vi "FABR-Append Stimulus Queue.vi"(0 "Runtime in":T2, 7 "SCL in":cluster{T1[]}[](array[cluster]), 11 "error in (no error)":errorcluster) -> (4 "Runtime out":T2, 8 "SCL out":cluster{T1[]}[](array[cluster]), 15 "error out":errorcluster)   [LabVIEW 2020]
uses:
  Typedefs/FABR-Runtime Data.ctl
  Typedefs/FABR-Stimulus Ticket.ctl
  Typedefs/FABR-Order.ctl
  Typedefs/FABR-Stimulus Condition.ctl
  debe6c45-fa08-4a77-9124-1a41b649b6a5.vi
  epl-vi-lib/Utility VIs/Math VIs/Math-Uniform Random Number (I32, 1D).vi
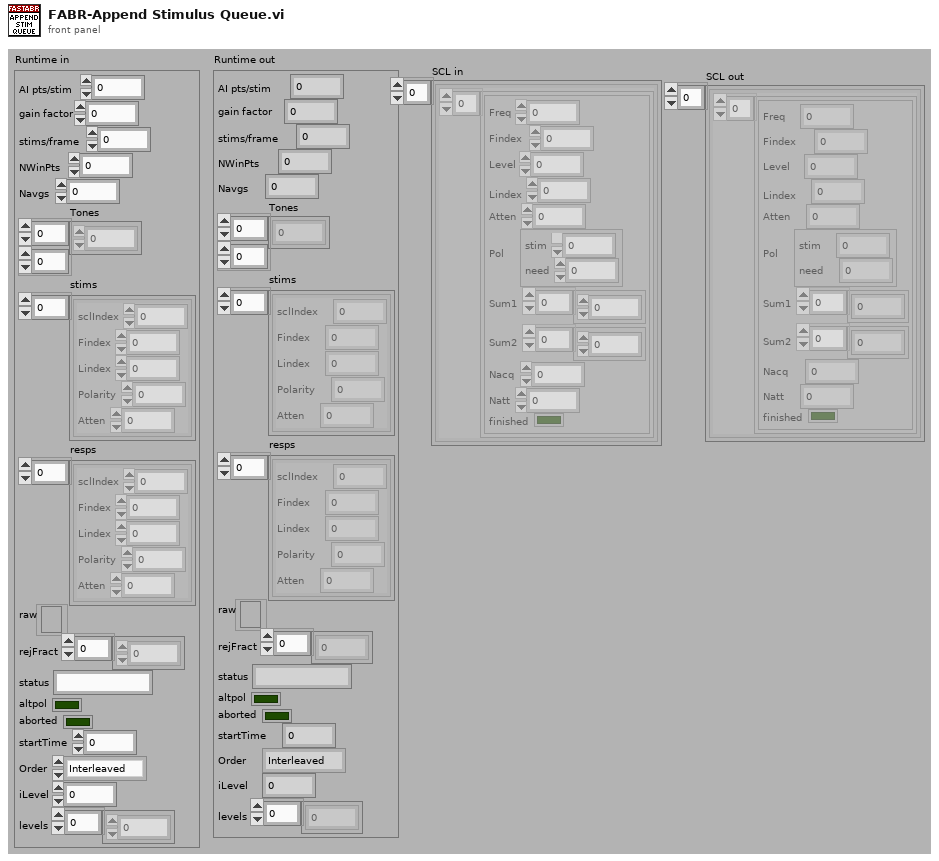
[diagram p1: front panel]
types:
  T1 = typedef "FABR-Stimulus Condition.ctl" = cluster{"Freq":dbl, "Findex":i32, "Level":dbl, "Lindex":i32, "Atten":dbl, "Pol":cluster{"stim":i32, "need":i32}, "Sum1":dbl[], "Sum2":dbl[], "Nacq":i32, "Natt":i32, "finished":bool}
  T2 = typedef "FABR-Runtime Data.ctl" = cluster{"AI pts/stim":i32, "gain factor":dbl, "stims/frame":i32, "NWinPts":i32, "Navgs":i32, "Tones":dbl[][], "stims":T3[], "resps":T3[], "raw":refnum<file>, "rejFract":dbl[], "status":string, "altpol":bool, "aborted":bool, "startTime":dbl, "Order":T4, "iLevel":i32, "levels":dbl[]}
  T3 = typedef "FABR-Stimulus Ticket.ctl" = cluster{"sclIndex":i32, "Findex":i32, "Lindex":i32, "Polarity":i32, "Atten":dbl}
  T4 = typedef "FABR-Order.ctl" = enum16{"Interleaved", "Stepped level"}
  T5 = cluster{i32, "Findex":i32, "Lindex":i32, "stim":i32, "Atten":dbl}
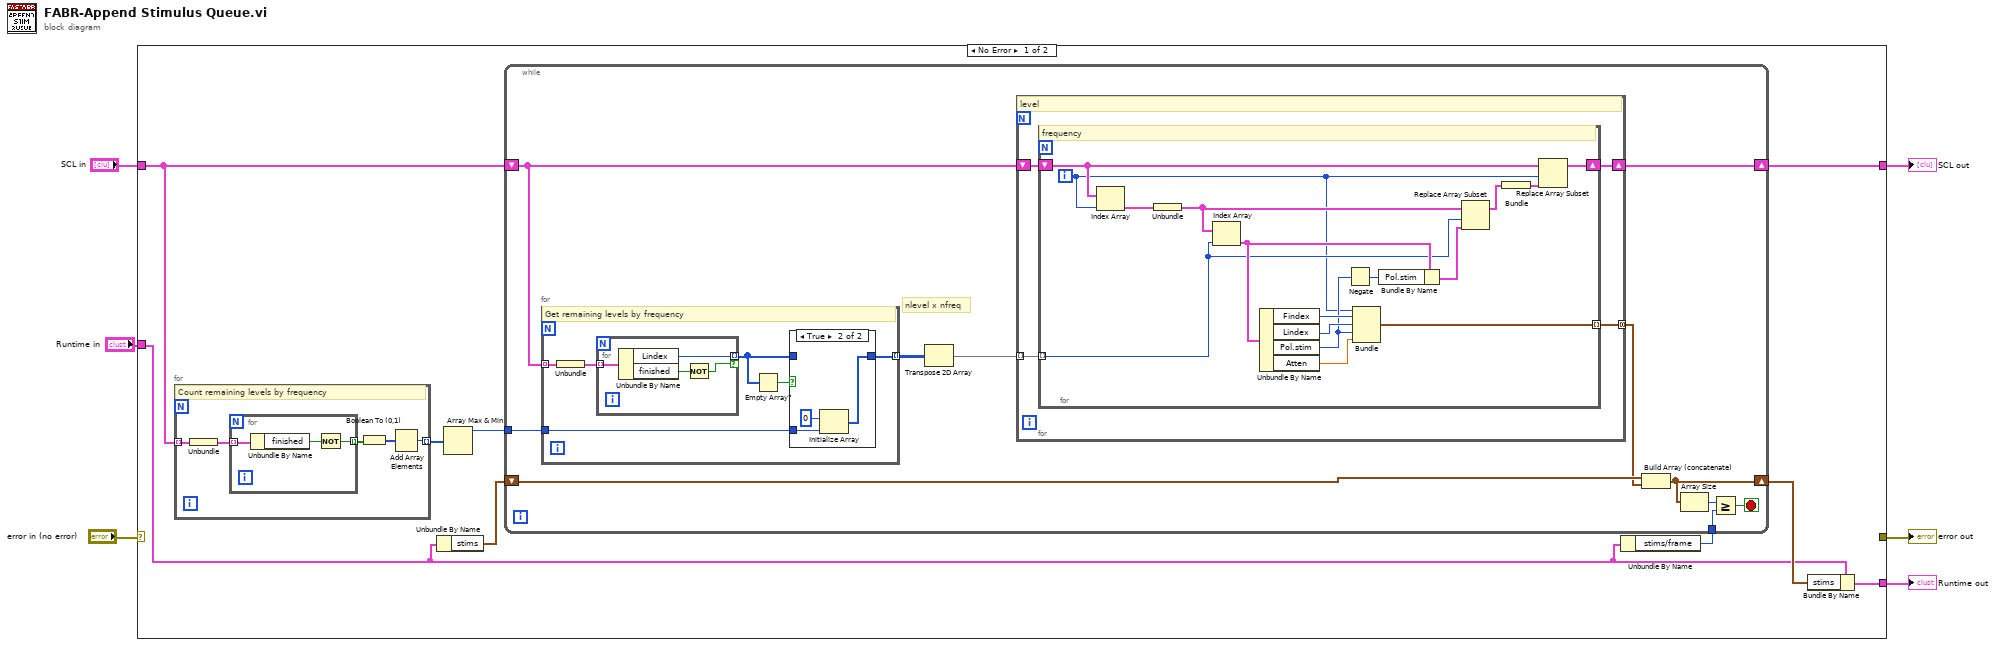
[diagram p0: block diagram]
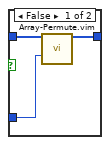
[diagram p2: hidden frame]
diagram:
  n1 = case shown="No Error" "error in (no error)" {
    selector: "error in (no error)" -> [_ w73]
    tunnel: [_ w73] -> w6
    tunnel: "Runtime in" -> [w8 w72]
    tunnel: [w13 w72] -> w4
    tunnel: "SCL in" -> [w14 w71]
    tunnel: [w12 w71] -> w1
    frame No Error {
      n2 = for {
        tunnel: w14 -> [w67] mode=indexing
        tunnel: [w63] -> w15 mode=indexing
        # "Count remaining levels by frequency"
        n3 = Unbundle(w67) -> (w66:T1[])
        n4 = for {
          tunnel: w66 -> [w70] mode=indexing
          tunnel: [w68] -> w64 mode=indexing
          n5 = Unbundle By Name(w70) -> ("finished"=w69:bool)
          n6 = Not(x=w69) -> (.not. x?=w68:bool)
        }
        n7 = Boolean To (0,1)(Boolean=w64) -> (0, 1=w65:i16[])
        n8 = Add Array Elements(numeric array=w65) -> (sum=w63:i16)
      }
      n9 = Unbundle By Name(w8) -> ("stims"=w10:T3[])
      n10 = Array Max & Min(array=w15) -> (max value=w11:i16)  [unwired: 3 out]
      n11 = Unbundle By Name(w8) -> ("stims/frame"=w7:i32)
      n12 = while {
        tunnel: w7 -> [w22]
        tunnel: w11 -> [w21]
        shift-right: [w23] -> w12
        shift-left: w14 -> [w25]
        shift-right: [w19] -> w9
        shift-left: w10 -> [w20]
        stop <- w16 stop-if-true
        # "nlevel x nfreq"
        n13 = for {
          tunnel: w25 -> [w52] mode=indexing
          tunnel: w21 -> [w50]
          tunnel: [w49] -> w26 mode=indexing
          # "Get remaining levels by frequency"
          n14 = Unbundle(w52) -> (w51:T1[])
          n15 = for {
            tunnel: w51 -> [w62] mode=indexing
            tunnel: [w60] -> w48 mode=indexing if=w59
            n16 = Unbundle By Name(w62) -> ("Lindex"=w60:i32, "finished"=w61:bool)
            n17 = Not(x=w61) -> (.not. x?=w59:bool)
          }
          n18 = Empty Array?(array=w48) -> (empty?=w47:bool)
          n19 = case shown="True" w47 {
            tunnel: w50 -> [w55 w58]
            tunnel: [w54 w56] -> w49
            tunnel: w48 -> [w53 _]
            frame False {
              n20 = call "Array-Permute.vim"("Array in"=w53, "N"=w55) -> ("Array out"=w54:i32[])  [unwired: 13 in]
            }
            frame True {
              n21 = Initialize Array(0, w58) -> (w56:i32[])
            }
          }
        }
        n22 = Transpose 2D Array(2D array=w26) -> (transposed array=w24:i32[][])
        n23 = for {
          tunnel: w24 -> [w29] mode=indexing
          tunnel: [w28] -> w18 mode=concatenating
          shift-right: [w27] -> w23
          shift-left: w25 -> [w30]
          # "level"
          n24 = for {
            tunnel: w29 -> [w39] mode=indexing
            tunnel: [w45] -> w28 mode=indexing
            shift-right: [w33] -> w27
            shift-left: w30 -> [w34]
            i -> [w31]
            # "frequency"
            n25 = Index Array(array=w34, index=w31) -> (element=w35:cluster{T1[]})
            n26 = Unbundle(w35) -> (w37:T1[])
            n27 = Index Array(array=w37, index=w39) -> (element=w42:T1)
            n28 = Unbundle By Name(w42) -> ("Findex"=w43:i32, "Lindex"=w46:i32, "Pol.stim"=w40:i32, "Atten"=w44:dbl)
            n29 = Negate(x=w40) -> (-x=w41:i32)
            n30 = Bundle(w31, "Findex"=w43, "Lindex"=w46, "stim"=w40, "Atten"=w44) -> (w45:T5)  [unwired: 1 in]
            n31 = Bundle By Name(cluster=w42, "Pol.stim"=w41) -> (w38:T1)
            n32 = Replace Array Subset(array=w37, new element=w38, index=w39) -> (w36:T1[])
            n33 = Bundle(w36) -> (w32:cluster{T1[]})  [unwired: 1 in]
            n34 = Replace Array Subset(array=w34, new element=w32, index=w31) -> (w33:cluster{T1[]}[])
          }
        }
        n35 = Build Array (concatenate)(w20, w18) -> (w19:T3[])
        n36 = Array Size(array=w19) -> (size(s)=w17:i32)
        n37 = Greater Or Equal?(x=w17, y=w22) -> (x >= y?=w16:bool)
      }
      n38 = Bundle By Name(cluster=w8, "stims"=w9) -> (w13:T2)
    }
    frame Error {
    }
  }
  "error out" <- w6
  "Runtime out" <- w4
  "SCL out" <- w1
